vi "Directional Speed Sensor Page.vi"(8 "error in (no error)":errorcluster, 11 "Node Ptr":T1 format="%.0x") -> (0 "error out":errorcluster)   [LabVIEW 2015, in "Engine Simulation Toolkit System Explorer.lvlib"]
uses:
  Engine Simulation Toolkit System Explorer.lvlib
  <vilib>/NI Veristand/Custom Device API/Custom Device Item Ref.ctl
  Shared/Properties.vi
  Shared/Constants and GUIDs.vi
  <vilib>/NI Veristand/Custom Device API/Get Item Property (Dependent Node Pointer).vi
  <vilib>/NI Veristand/Custom Device API/Get Item Property (String).vi
  <vilib>/NI Veristand/Custom Device Tools/Custom Device Utility Library/NI VeriStand - Search for All Items by GUID.vi
  <vilib>/NI Veristand/Custom Device API/Set Item Property (Dependent Node Pointer).vi
  <vilib>/NI Veristand/Custom Device API/Custom Device API.lvlib
  Shared/Engine Simulation Toolkit Shared.lvlib
  <vilib>/NI Veristand/Custom Device Tools/Custom Device Utility Library/Custom Device Utility Library.lvlib
panel:
  in  "ToothSource":u16(ring) caption="Digital pattern to use for tooth centers"
  in  "Tr (uS)":dbl min=0.0 max=1638.4 step=0.025
  in  "Tf (uS)":dbl min=0.0 max=1638.4 step=0.025
  in  "Td (uS)":dbl min=0.0 max=1638.4 step=0.025
  out "Name in bitfile":string
  in  "Name":string
  in  "Header":cluster{"Section Name":string}={"Section Name"="Directional Speed Sensor Settings"}
  # "(Delay time)"
  # "(Forward pulse duration)"
  # "(Reverse pulse duration)"
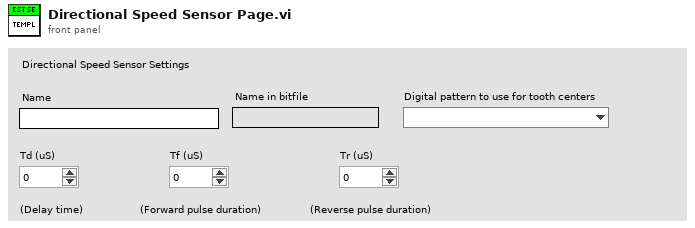
[diagram p1: front panel]
types:
  T1 = typedef "Custom Device API.lvlib/Custom Device Item Ref.ctl" = u64
  T2 = typedef "Engine Simulation Toolkit Shared.lvlib/Channel.ctl" = cluster{"Name":string, "Units":string, "Default":dbl, "Description":string}
  T3 = typedef "Custom Device API.lvlib/Custom Device Item Info.ctl" = cluster{"Name":string, "Is Channel":bool, "GUID":string, "Is Waveform":bool}
  T4 = typedef "Custom Device API.lvlib/Custom Device Commands.ctl" = enum16{"Default", "Item renamed", "Shutdown", "Dynamic button pressed"}
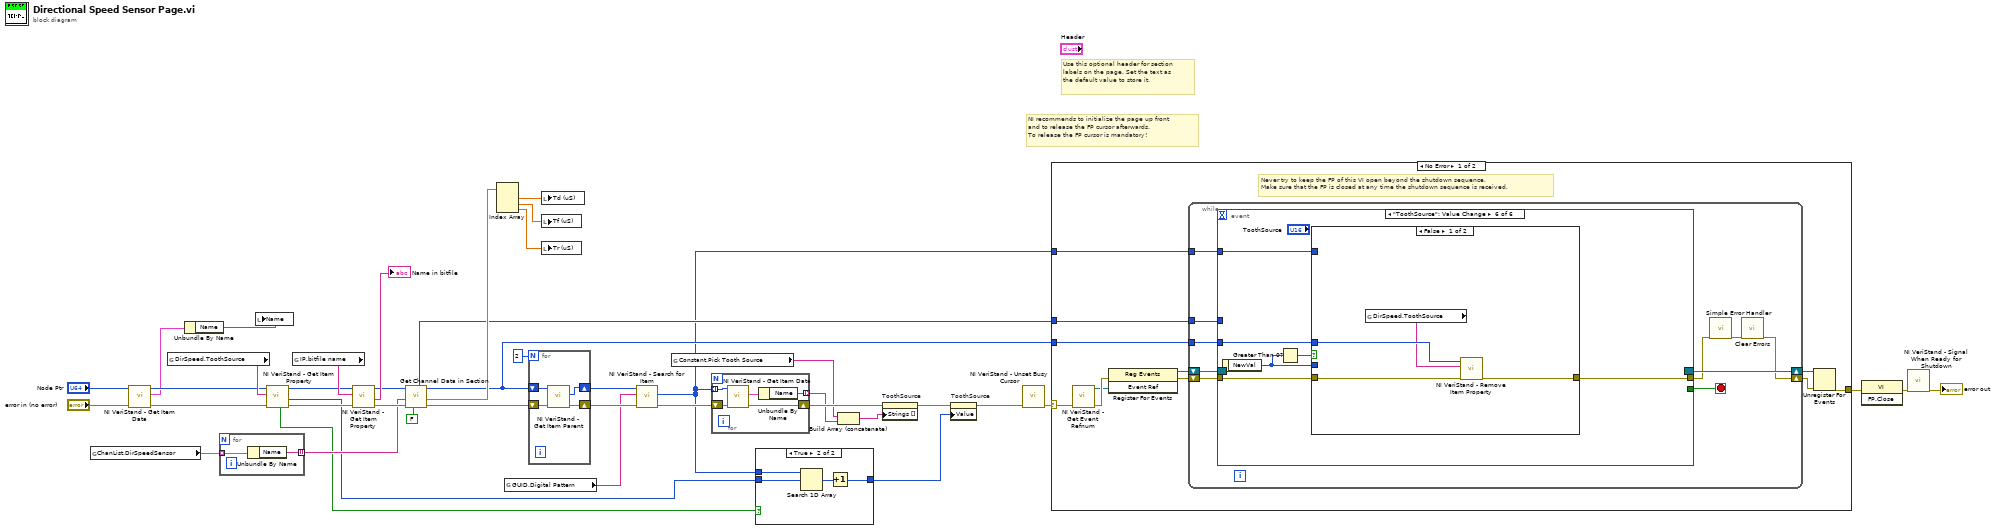
[diagram p0: block diagram]
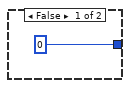
[diagram p2: hidden frame]
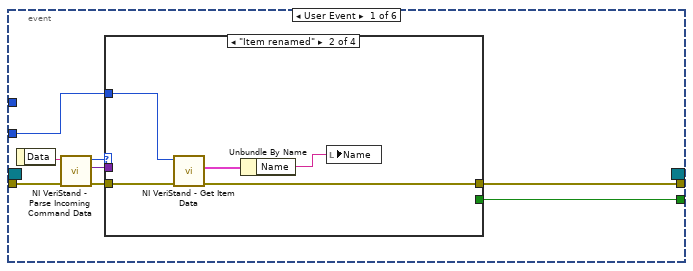
[diagram p3: hidden frame]
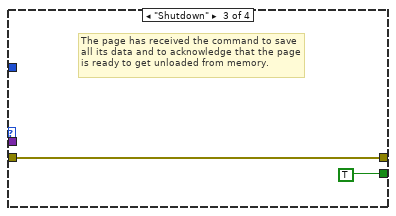
[diagram p5: hidden frame]
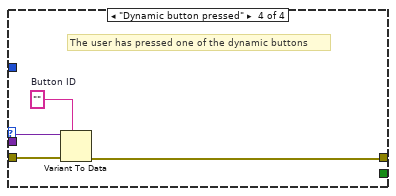
[diagram p6: hidden frame]
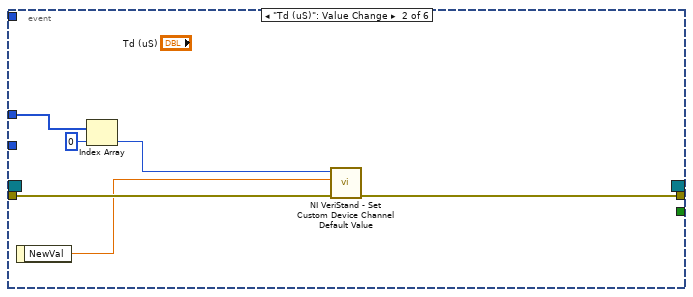
[diagram p7: hidden frame]
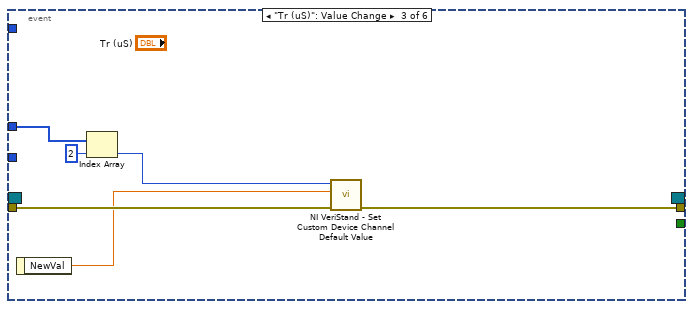
[diagram p8: hidden frame]
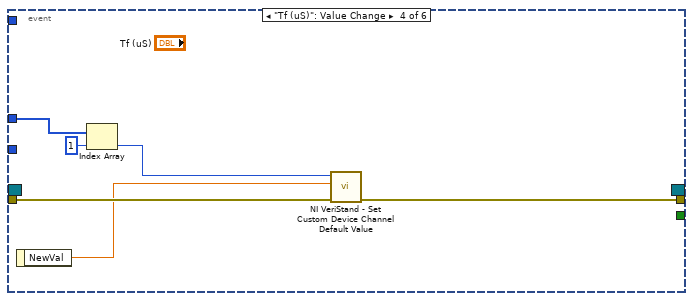
[diagram p9: hidden frame]
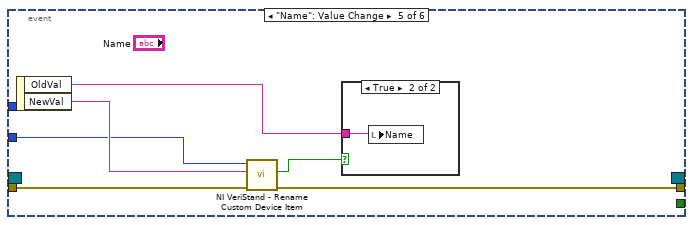
[diagram p10: hidden frame]
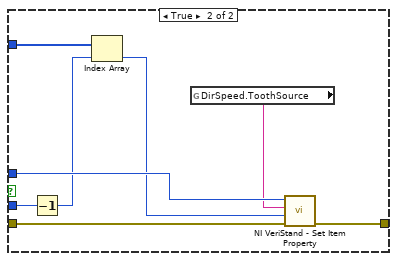
[diagram p12: hidden frame]
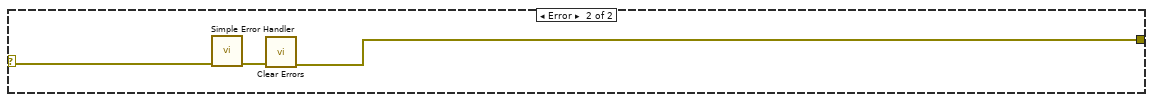
[diagram p13: hidden frame]
diagram:
  # "Use this optional header for section labels on the page. Set the text as the default value to store it."
  # "NI recommends to initialize the page up front\nand to release the FP cursor afterwards.\nTo release the FP cursor is mandatory!"
  n1 = global read "Constants and GUIDs.vi" "ChanList.DirSpeedSensor"() -> (w32:T2[])
  n2 = call <vilib>:"NI VeriStand - Get Item Data.vi"("error in (no error)"="error in (no error)", "Item Ref in"="Node Ptr") -> ("error out"=w5:errorcluster, "Item Info"=w2:T3, "Item Ref out"=w3:T1)  [unwired: 6 in, 1 out]
  n3 = global read "Properties.vi" "DirSpeed.ToothSource"() -> (w16:string)
  n4 = Unbundle By Name(w2) -> ("Name"=w1:string)
  n5 = for {
    tunnel: w32 -> [w44] mode=indexing
    tunnel: [w43] -> w31 mode=indexing
    n6 = Unbundle By Name(w44) -> ("Name"=w43:string)
  }
  n7 = local write "Name"(w1) -> ()
  n8 = call-poly <vilib>:"NI VeriStand - Get Item Property.vi"("error in (no error)"=w5, "Property Name"=w16, "Item Ref in"=w3) -> ("error out"=w18:errorcluster, "Dependent Node Ref"=w7:T1, "Item Ref out"=w17:T1, "Found"=w9:bool)  [unwired: 5 in]
  n9 = global read "Properties.vi" "IP.bitfile name"() -> (w37:string)
  n10 = call-poly <vilib>:"NI VeriStand - Get Item Property.vi"("error in (no error)"=w18, "Property Name"=w37, "Item Ref in"=w17) -> ("error out"=w35:errorcluster, "Value"=→"Name in bitfile":string, "Item Ref out"=w33:T1)  [unwired: 5 in, 1 out]
  n11 = call "Get Channel Data in Section.vi"("Get FIFO indexes (T)"=FALSE, "error in (no error)"=w35, "Channels"=w31, "Item Ref in"=w33) -> ("error out"=w34:errorcluster, "default values"=w29:dbl[], "Item Ref out"=w23:T1, "channel refs"=w25:T1[])  [unwired: 3 in, 1 out]
  n12 = Index Array(array=w29) -> (element #1=w28:dbl, element #2=w27:dbl, element #3=w26:dbl)  [unwired: 3 in]
  n13 = global read "Constants and GUIDs.vi" "GUID.Digital Pattern"() -> (w19:string)
  n14 = for {
    N: 2 -> [_]
    shift-right: [w45] -> w20
    shift-left: w23 -> [w46]
    shift-right: [w47] -> w24
    shift-left: w34 -> [w48]
    n15 = call <vilib>:"NI VeriStand - Get Item Parent.vi"("error in (no error)"=w48, "Item Ref in"=w46) -> ("error out"=w47:errorcluster, "Parent Ref"=w45:T1)  [unwired: 6 in, 2 out]
  }
  n16 = local write "Td (uS)"(w28) -> ()
  n17 = local write "Tf (uS)"(w27) -> ()
  n18 = local write "Tr (uS)"(w26) -> ()
  n19 = call-poly <vilib>:"NI VeriStand - Search for Item.vi"("error in"=w24, "Item GUID"=w19, "Section Ref in"=w20) -> ("error out"=w21:errorcluster, "Item Refs"=w6:T1[])  [unwired: 5 in, 2 out]
  n20 = global read "Constants and GUIDs.vi" "Constant.Pick Tooth Source"() -> (w10:string)
  n21 = for {
    shift-right: [w52] -> w15
    shift-left: w21 -> [w53]
    tunnel: w6 -> [w51] mode=indexing
    tunnel: [w49] -> w14 mode=indexing
    n22 = call <vilib>:"NI VeriStand - Get Item Data.vi"("error in (no error)"=w53, "Item Ref in"=w51) -> ("error out"=w52:errorcluster, "Item Info"=w50:T3)  [unwired: 6 in, 2 out]
    n23 = Unbundle By Name(w50) -> ("Name"=w49:string)
  }
  n24 = case shown="True" w9 {
    tunnel: w6 -> [_ w58]
    tunnel: [0 w56] -> w8
    tunnel: w7 -> [_ w55]
    frame False {
    }
    frame True {
      n25 = Search 1D Array(1D array=w58, element=w55) -> (index of element=w57:i32)  [unwired: 1 in]
      n26 = Increment(x=w57) -> (x+1=w56:i32)
    }
  }
  n27 = Build Array (concatenate)(w10, w14) -> (w11:string[])
  n28 = property on="ToothSource" class="Ring (strict)"(error in=w15, "Strings []"=w11) -> (error out=w13:errorcluster)  [unwired: 1 in, 1 out]
  n29 = property on="ToothSource" class="Ring (strict)"(error in=w13, "Value"=w8) -> (error out=w12:errorcluster)  [unwired: 1 in, 1 out]
  n30 = call <vilib>:"NI VeriStand - Unset Busy Cursor.vi"("error in (no error)"=w12) -> ("error out"=w39:errorcluster)  [unwired: 10 out]
  n31 = case shown="No Error" w39 {
    selector: w39 -> [w61 w145]
    tunnel: [w66 w143] -> w42
    tunnel: w23 -> [w62 _]
    tunnel: w25 -> [w60 _]
    tunnel: w6 -> [w59 _]
    frame No Error {
      # "Never try to keep the FP of this VI open beyond the shutdown sequence.\nMake sure that the FP is closed at any time the shutdown sequence is received."
      n32 = call <vilib>:"NI VeriStand - Get Event Refnum.vi"("error in (no error)"=w61) -> ("error out"=w69:errorcluster, "Event Ref"=w65:refnum<user-event>)  [unwired: 9 out]
      n33 = register-events(error in=w69, w65) -> (reference out=w63:refnum<event-registration>, error out=w64:errorcluster)  [unwired: 1 in]
      n34 = while {
        tunnel: w62 -> [w75]
        shift-right: [w72] -> w67
        shift-left: w64 -> [w78]
        shift-right: [w79] -> w68
        shift-left: w63 -> [w77]
        tunnel: w60 -> [w71]
        tunnel: w59 -> [w70]
        stop <- w76 stop-if-true
        n35 = event shown="[5] \"ToothSource\": Value Change" {
          selector: w77 -> [_ _ _ _ _ _]
          dyn-events: [_ _ _ _ _ _] -> w79
          timeout: _ -> [_ _ _ _ _ _]
          tunnel: w78 -> [w87 w105 w111 w117 w123 w130]
          tunnel: [w83 _ _ _ _ _] -> w76
          tunnel: [w82 w104 w110 w116 w122 w129] -> w74
          tunnel: w75 -> [w81 _ _ _ w120 w128]
          tunnel: w71 -> [_ w102 w108 w114 _ _]
          tunnel: w70 -> [_ _ _ _ _ w127]
          event User Event {
            n36 = event-data() -> ("Data"=w86:string)  [unwired: 1 out]
            n37 = call <vilib>:"NI VeriStand - Parse Incoming Command Data.vi"("error in (no error)"=w87, "Incoming data"=w86) -> ("error out"=w85:errorcluster, "Outgoing data"=w80:variant, "Action"=w84:T4)  [unwired: 7 out]
            n38 = case shown="\"Item renamed\"" w84 {
              tunnel: w85 -> [w88 w92 w94 w99]
              tunnel: [_ _ TRUE _] -> w83
              tunnel: [w88 w90 w94 w96] -> w82
              tunnel: w81 -> [_ w91 _ _]
              tunnel: w80 -> [_ _ _ w98]
              frame "Default", Default {
              }
              frame "Item renamed" {
                n39 = call <vilib>:"NI VeriStand - Get Item Data.vi"("error in (no error)"=w92, "Item Ref in"=w91) -> ("error out"=w90:errorcluster, "Item Info"=w93:T3)  [unwired: 8 out]
                n40 = Unbundle By Name(w93) -> ("Name"=w89:string)
                n41 = local write "Name"(w89) -> ()
              }
              frame "Shutdown" {
                # "The page has received the command to save all its data and to acknowledge that the page is ready to get unloaded from memory."
              }
              frame "Dynamic button pressed" {
                w97 = ""  # Button ID
                # "The user has pressed one of the dynamic buttons"
                n42 = Variant To Data(error in=w99, type=w97, Variant=w98) -> (error out=w96:errorcluster)  [unwired: 1 out]
              }
            }
          }
          event "Td (uS)": Value Change {
            n43 = event-data() -> ("NewVal"=w103:dbl)  [unwired: 1 out]
            n44 = Index Array(array=w102, index=0) -> (element=w101:T1)
            n45 = call <vilib>:"NI VeriStand - Set Custom Device Channel Default Value.vi"("error in (no error)"=w105, "Default Value"=w103, "Channel Ref in"=w101) -> ("error out"=w104:errorcluster)  [unwired: 7 in, 1 out]
          }
          event "Tr (uS)": Value Change {
            n46 = event-data() -> ("NewVal"=w109:dbl)  [unwired: 1 out]
            n47 = Index Array(array=w108, index=2) -> (element=w107:T1)
            n48 = call <vilib>:"NI VeriStand - Set Custom Device Channel Default Value.vi"("error in (no error)"=w111, "Default Value"=w109, "Channel Ref in"=w107) -> ("error out"=w110:errorcluster)  [unwired: 7 in, 1 out]
          }
          event "Tf (uS)": Value Change {
            n49 = event-data() -> ("NewVal"=w115:dbl)  [unwired: 1 out]
            n50 = Index Array(array=w114, index=1) -> (element=w113:T1)
            n51 = call <vilib>:"NI VeriStand - Set Custom Device Channel Default Value.vi"("error in (no error)"=w117, "Default Value"=w115, "Channel Ref in"=w113) -> ("error out"=w116:errorcluster)  [unwired: 7 in, 1 out]
          }
          event "Name": Value Change {
            n52 = event-data() -> ("OldVal"=w118:string, "NewVal"=w121:string)  [unwired: 1 out]
            n53 = call <vilib>:"NI VeriStand - Rename Custom Device Item.vi"("error in (no error)"=w123, "New Name"=w121, "Item Ref in"=w120) -> ("error out"=w122:errorcluster, "Request invalid?"=w119:bool)  [unwired: 1 in, 6 out]
            n54 = case shown="True" w119 {
              tunnel: w118 -> [_ w124]
              frame False {
              }
              frame True {
                n55 = local write "Name"(w124) -> ()
              }
            }
          }
          event "ToothSource": Value Change {
            n56 = event-data() -> ("NewVal"=w125:u16)  [unwired: 1 out]
            n57 = Greater Than 0?(x=w125) -> (x > 0?=w126:bool)
            n58 = case shown="False" w126 {
              tunnel: w130 -> [w134 w142]
              tunnel: [w133 w141] -> w129
              tunnel: w128 -> [w132 w140]
              tunnel: w125 -> [_ w139]
              tunnel: w127 -> [_ w138]
              frame False {
                n59 = global read "Properties.vi" "DirSpeed.ToothSource"() -> (w131:string)
                n60 = call <vilib>:"NI VeriStand - Remove Item Property.vi"("error in (no error)"=w134, "Property Name"=w131, "Item Ref in"=w132) -> ("error out"=w133:errorcluster)  [unwired: 6 in, 2 out]
              }
              frame True {
                n61 = Decrement(x=w139) -> (x-1=w137:u16)
                n62 = Index Array(array=w138, index=w137) -> (element=w136:T1)
                n63 = global read "Properties.vi" "DirSpeed.ToothSource"() -> (w135:string)
                n64 = call-poly <vilib>:"NI VeriStand - Set Item Property.vi"("error in (no error)"=w142, "Dependent Node Ref"=w136, "Property Name"=w135, "Item Ref in"=w140) -> ("error out"=w141:errorcluster)  [unwired: 5 in, 2 out]
              }
            }
          }
        }
        n65 = call <vilib>:"Simple Error Handler.vi"("error in (no error)"=w74) -> ("error out"=w73:errorcluster)  [unwired: 1 in, 7 out]
        n66 = call <vilib>:"Clear Errors.vi"("error in (no error)"=w73) -> ("error out"=w72:errorcluster)  [unwired: 1 in, 5 out]
      }
      n67 = Unregister For Events(event registration refnum=w68, error in=w67) -> (error out=w66:errorcluster)
    }
    frame Error {
      n68 = call <vilib>:"Simple Error Handler.vi"("error in (no error)"=w145) -> ("error out"=w144:errorcluster)  [unwired: 1 in, 7 out]
      n69 = call <vilib>:"Clear Errors.vi"("error in (no error)"=w144) -> ("error out"=w143:errorcluster)  [unwired: 1 in, 5 out]
    }
  }
  n70 = invoke class="VI" method="FP.Close"(error in=w42) -> (error out=w41:errorcluster)  [unwired: 2 in, 2 out]
  n71 = call <vilib>:"NI VeriStand - Signal When Ready for Shutdown.vi"("error in (no error)"=w41) -> ("error out"=→"error out":errorcluster)  [unwired: 10 out]
